vi "Q4.vi"() -> ()   [LabVIEW 2014]
panel:
  out "number":i32
  out "debug array":dbl[](array[numeric])
  out "Array":i32[][](array[numeric])
  in  "stairs":i32
  # "可行方案數"
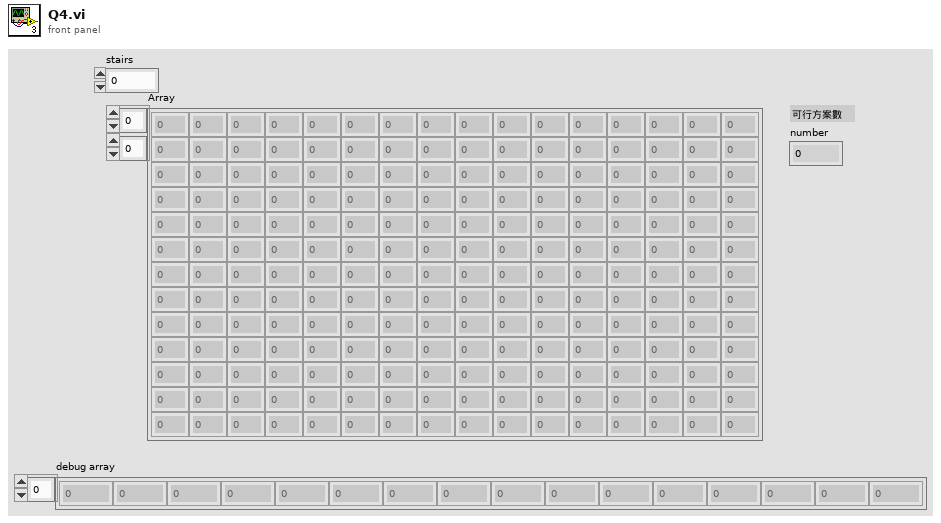
[diagram p1: front panel]
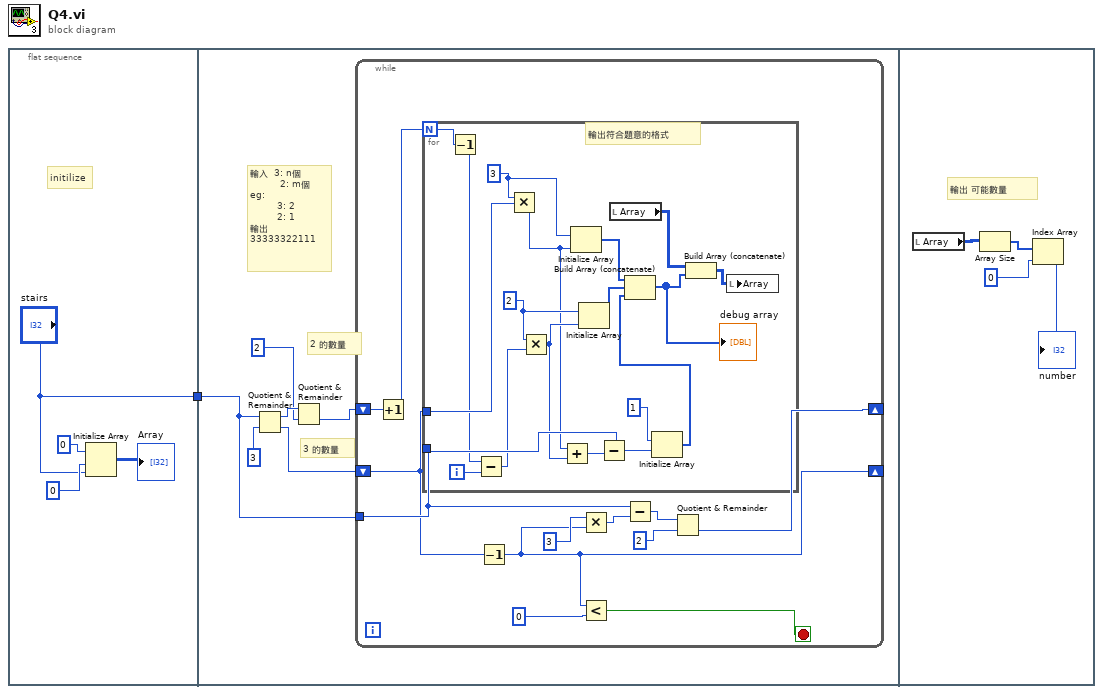
[diagram p0: block diagram]
diagram:
  n1 = flat-sequence {
    tunnel: ["stairs"] -> w1
    tunnel: w1 -> [w8]
    frame #0 {
      # "initilize"
      n2 = Initialize Array(0, 0, "stairs") -> (→"Array":i32[][])
    }
    frame #1 {
      # "輸入  3: n個\n          2: m個\neg: \n         3: 2 \n         2: 1\n輸出 33333322111"
      # "3 的數量"
      # "2 的數量"
      n3 = Quotient & Remainder(x=w8, y=3) -> (x-y*floor(x/y)=w10:i32, floor(x/y)=w9:i32)
      n4 = Quotient & Remainder(x=w10, y=2) -> (floor(x/y)=w6:i32)  [unwired: 1 out]
      n5 = while {
        shift-right: [w13] -> _
        shift-left: w6 -> [w12]
        shift-right: [w17] -> _
        shift-left: w9 -> [w14]
        tunnel: w8 -> [w15]
        stop <- w22 stop-if-true
        n6 = Increment(x=w12) -> (x+1=w16:i32)
        n7 = for {
          N: w16 -> [w29]
          tunnel: w14 -> [w42]
          tunnel: w15 -> [w38]
          i -> [w30]
          w39 = 2
          w33 = 3
          # "輸出符合題意的格式"
          n8 = Decrement(x=w29) -> (x-1=w27:i32)
          n9 = Subtract(x=w27, y=w30) -> (x-y=w28:i32)
          n10 = Multiply(x=w33, y=w42) -> (x*y=w31:i32)
          n11 = Multiply(x=w39, y=w28) -> (x*y=w32:i32)
          n12 = Add(x=w31, y=w32) -> (x+y=w37:i32)
          n13 = Initialize Array(w33, w31) -> (w41:i32[])
          n14 = Initialize Array(w39, w32) -> (w40:i32[])
          n15 = Subtract(x=w38, y=w37) -> (x-y=w36:i32)
          n16 = local read "Array"() -> (w26:i32[][])
          n17 = Initialize Array(1, w36) -> (w34:i32[])
          n18 = Build Array (concatenate)(w41, w40, w34) -> (w25:i32[])
          "debug array" <- w25
          n19 = Build Array (concatenate)(w26, w25) -> (w24:i32[][])
          n20 = local write "Array"(w24) -> ()
        }
        n21 = Decrement(x=w14) -> (x-1=w17:i32)
        n22 = Multiply(x=3, y=w17) -> (x*y=w20:i32)
        n23 = Less?(x=w17, y=0) -> (x < y?=w22:bool)
        n24 = Subtract(x=w15, y=w20) -> (x-y=w19:i32)
        n25 = Quotient & Remainder(x=w19, y=2) -> (floor(x/y)=w13:i32)  [unwired: 1 out]
      }
    }
    frame #2 {
      # "輸出 可能數量"
      n26 = local read "Array"() -> (w46:i32[][])
      n27 = Array Size(array=w46) -> (size(s)=w45:i32[])
      n28 = Index Array(array=w45, index=0) -> (element=→"number":i32)
    }
  }
